vi "HM8118 - Configure Signal.vi"(7 "Frequency (1kHz)":dbl=1000.0 min=20.0 max=200000.0, 8 "error in (no error)":errorcluster, 10 "Measuring Voltage (1V)":dbl=1.0 min=0.05 max=1.5 step=0.01, 11 "VISA resource name":refnum<visa-resource-name>) -> (0 "error out":errorcluster, 3 "VISA resource name out":refnum<visa-resource-name>)   [LabVIEW 2017]
doc: "Configures the voltage level and frequency of the measurement signal."
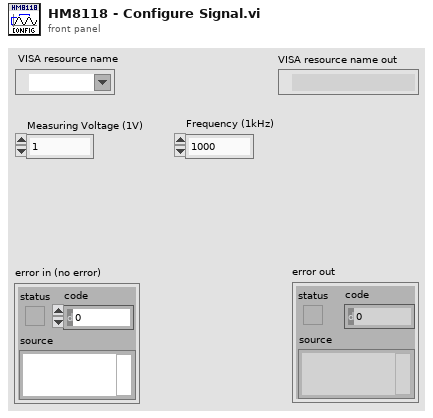
[diagram p1: front panel]
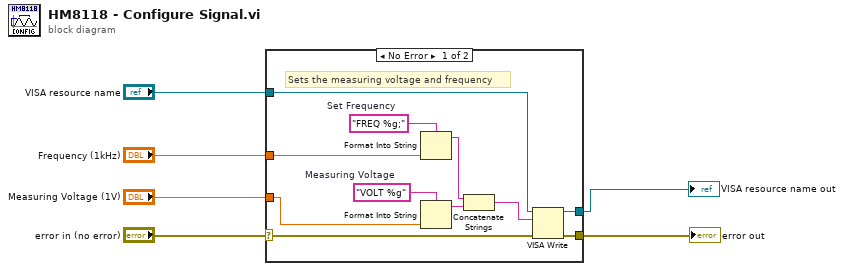
[diagram p0: block diagram]
diagram:
  n1 = case shown="No Error" "error in (no error)" {
    selector: "error in (no error)" -> [w7 w19]
    tunnel: "VISA resource name" -> [w17 w18]
    tunnel: "Frequency (1kHz)" -> [w12 _]
    tunnel: "Measuring Voltage (1V)" -> [w10 _]
    tunnel: [w9 w18] -> w3
    tunnel: [w8 w19] -> w2
    frame No Error {
      w15 = "VOLT %g"  # Measuring Voltage
      w16 = "FREQ %g;"  # Set Frequency
      # "Sets the measuring voltage and frequency"
      n2 = Format Into String(format string=w16, w12) -> (resulting string=w11:string)  [unwired: 2 in, 1 out]
      n3 = Format Into String(format string=w15, w10) -> (resulting string=w14:string)  [unwired: 2 in, 1 out]
      n4 = Concatenate Strings(w11, w14) -> (w13:string)
      n5 = VISA Write(VISA resource name=w17, write buffer=w13, error in (no error)=w7) -> (VISA resource name out=w9:refnum<visa-resource-name>, error out=w8:errorcluster)  [unwired: 1 out]
    }
    frame Error {
    }
  }
  "error out" <- w2
  "VISA resource name out" <- w3
